vi "All_Stages_Action.vi"(6 "Positions":dbl[](array[numeric]), 8 "Axis":bool[](array[boolean]), 9 "Action":T1=enum."MVR", 10 "Stage ID":string, 11 "State Cluster":T2={"Stages"={"M686"={"VISA"="", "Status"=FALSE, "Positions"=[], "SpecialFunction"="", "ID"="M686"}, "P541"={"VISA"="", "Status"=FALSE, "Positions"=[], "SpecialFunction"="", "ID"="P541"}, "M227"={"VISA"="", "Status"=FALSE, "Positions"=[], "SpecialFunction"="", "ID"="M227"}, "N664"={"VISA"="", "Status"=FALSE, "Positions"=[], "SpecialFunction"="", "ID"="N664"}, "P612"={"VISA"="", "Status"=FALSE, "Positions"=[], "SpecialFunction"="", "ID"="P612"}, "ASI"={"VISA"="", "Status"=FALSE, "Positions"=[], "SpecialFunction"="", "ID"="ASI"}}, "Lasers"={"405"={"VISA"=""}, "561"={"handle"=0, "Return Value"=0}}}) -> (0 "Position Out":dbl[](array[numeric]), 3 "State Cluster Out":T2={"Stages"={"M686"={"VISA"="", "Status"=FALSE, "Positions"=[], "SpecialFunction"="", "ID"="M686"}, "P541"={"VISA"="", "Status"=FALSE, "Positions"=[], "SpecialFunction"="", "ID"="P541"}, "M227"={"VISA"="", "Status"=FALSE, "Positions"=[], "SpecialFunction"="", "ID"="M227"}, "N664"={"VISA"="", "Status"=FALSE, "Positions"=[], "SpecialFunction"="", "ID"="N664"}, "P612"={"VISA"="", "Status"=FALSE, "Positions"=[], "SpecialFunction"="", "ID"="P612"}, "ASI"={"VISA"="", "Status"=FALSE, "Positions"=[], "SpecialFunction"="", "ID"="ASI"}}, "Lasers"={"405"={"VISA"=""}, "561"={"handle"=0, "Return Value"=0}}})   [LabVIEW 2014]
uses:
  Controls/State_Cluster.ctl
  iPALM Control/Controls/StageStates.ctl
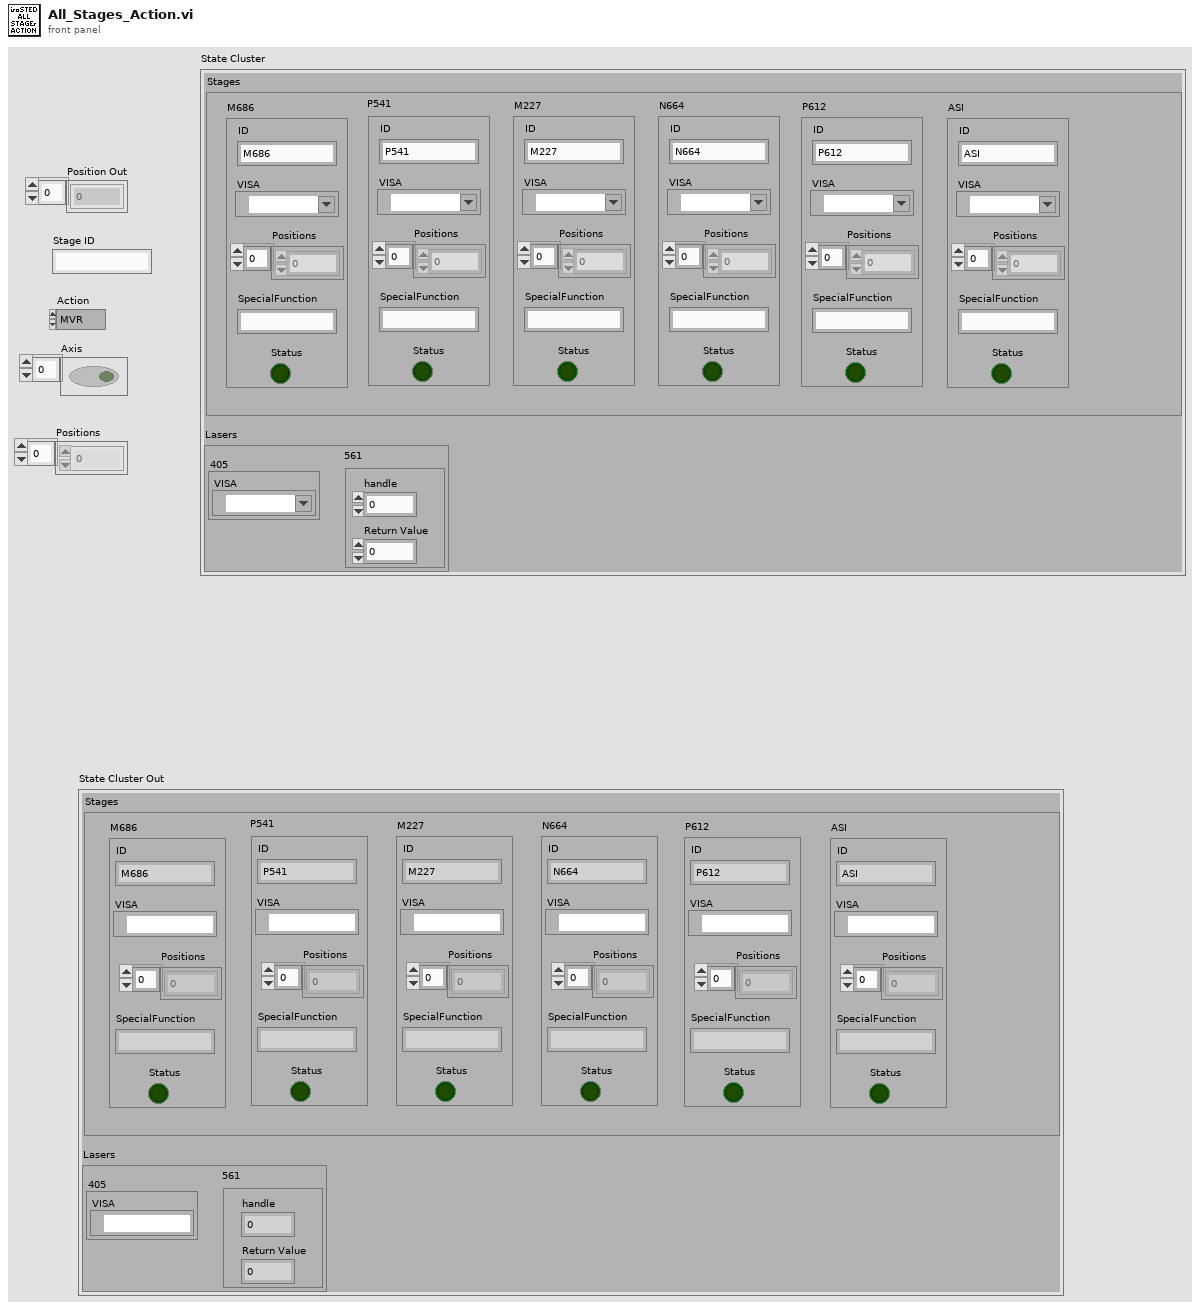
[diagram p1: front panel]
types:
  T1 = typedef "StageStates.ctl" = enum16{"POSITION", "MVR", "MOVE", "HALT", "ONTARGET", "ERROR", "EXIT", "HOME", "ZEROPOS", "NANOPOS", "QUIT", "ANALOG"}
  T2 = typedef "State_Cluster.ctl" = cluster{"Stages":cluster{"M686":cluster{"VISA":refnum<visa-resource-name>, "Status":bool, "Positions":dbl[], "SpecialFunction":string, "ID":string}, "P541":cluster{"VISA":refnum<visa-resource-name>, "Status":bool, "Positions":dbl[], "SpecialFunction":string, "ID":string}, "M227":cluster{"VISA":refnum<visa-resource-name>, "Status":bool, "Positions":dbl[], "SpecialFunction":string, "ID":string}, "N664":cluster{"VISA":refnum<visa-resource-name>, "Status":bool, "Positions":dbl[], "SpecialFunction":string, "ID":string}, "P612":cluster{"VISA":refnum<visa-resource-name>, "Status":bool, "Positions":dbl[], "SpecialFunction":string, "ID":string}, "ASI":cluster{"VISA":refnum<visa-resource-name>, "Status":bool, "Positions":dbl[], "SpecialFunction":string, "ID":string}}, "Lasers":cluster{"405":cluster{"VISA":refnum<visa-resource-name>}, "561":cluster{"handle":u32, "Return Value":i32}}}
  T3 = cluster{"M686":cluster{"VISA":refnum<visa-resource-name>, "Status":bool, "Positions":dbl[], "SpecialFunction":string, "ID":string}, "P541":cluster{"VISA":refnum<visa-resource-name>, "Status":bool, "Positions":dbl[], "SpecialFunction":string, "ID":string}, "M227":cluster{"VISA":refnum<visa-resource-name>, "Status":bool, "Positions":dbl[], "SpecialFunction":string, "ID":string}, "N664":cluster{"VISA":refnum<visa-resource-name>, "Status":bool, "Positions":dbl[], "SpecialFunction":string, "ID":string}, "P612":cluster{"VISA":refnum<visa-resource-name>, "Status":bool, "Positions":dbl[], "SpecialFunction":string, "ID":string}, "ASI":cluster{"VISA":refnum<visa-resource-name>, "Status":bool, "Positions":dbl[], "SpecialFunction":string, "ID":string}}
  T4 = cluster{"VISA":refnum<visa-resource-name>, "Status":bool, "Positions":dbl[], "SpecialFunction":string, "ID":string}[]
  T5 = cluster{"VISA":refnum<visa-resource-name>, "Status":bool, "Positions":dbl[], "SpecialFunction":string, "ID":string}
  T6 = cluster{"Stages[0]":cluster{"VISA":refnum<visa-resource-name>, "Status":bool, "Positions":dbl[], "SpecialFunction":string, "ID":string}, "Stages[1]":cluster{"VISA":refnum<visa-resource-name>, "Status":bool, "Positions":dbl[], "SpecialFunction":string, "ID":string}, "Stages[2]":cluster{"VISA":refnum<visa-resource-name>, "Status":bool, "Positions":dbl[], "SpecialFunction":string, "ID":string}, "Stages[3]":cluster{"VISA":refnum<visa-resource-name>, "Status":bool, "Positions":dbl[], "SpecialFunction":string, "ID":string}, "Stages[4]":cluster{"VISA":refnum<visa-resource-name>, "Status":bool, "Positions":dbl[], "SpecialFunction":string, "ID":string}, "Stages[5]":cluster{"VISA":refnum<visa-resource-name>, "Status":bool, "Positions":dbl[], "SpecialFunction":string, "ID":string}}
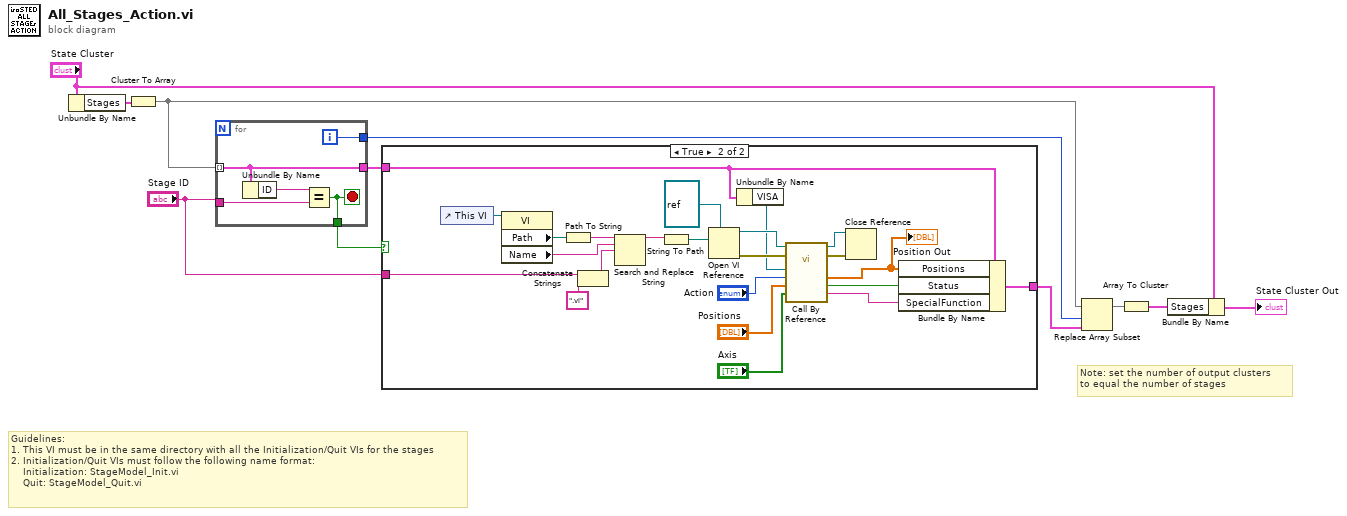
[diagram p0: block diagram]
diagram:
  # "Note: set the number of output clusters \nto equal the number of stages"
  # "Guidelines:\n1. This VI must be in the same directory with all the Initialization/Quit VIs for the stages\n2. Initialization/Quit VIs must follow the following name format:\n    Initialization: StageModel_Init.vi\n    Quit: StageModel_Quit.vi"
  n1 = Unbundle By Name("State Cluster") -> ("Stages"=w4:T3)
  n2 = Cluster To Array(cluster=w4) -> (array=w11:T4)
  n3 = for {
    tunnel: w11 -> [w15] mode=indexing
    tunnel: "Stage ID" -> [w16]
    tunnel: [w15] -> w6
    tunnel: [w14] -> w10
    tunnel: [w12] -> w7
    i -> [w14]
    stop <- w12 stop-if-true
    n4 = Unbundle By Name(w15) -> ("ID"=w13:string)
    n5 = Equal?(x=w13, y=w16) -> (x = y?=w12:bool)
  }
  n6 = case shown="True" w7 {
    tunnel: [w17 w35] -> w5
    tunnel: "Stage ID" -> [_ w36]
    tunnel: w6 -> [w17 w22]
    frame False {
    }
    frame True {
      n7 = control-ref of="This VI"() -> (w40:refnum<vi>)
      n8 = property class="VI"(reference=w40) -> ("Path"=w39:path, "Name"=w37:string)  [unwired: 1 in, 2 out]
      n9 = Path To String(path=w39) -> (string=w38:string)
      n10 = Concatenate Strings(w36, ".vi" ("string")) -> (w25:string)
      n11 = Search and Replace String(input string=w38, search string=w37, replace string=w25) -> (result string=w32:string)  [unwired: 5 in, 3 out]
      n12 = String To Path(string=w32) -> (path=w31:path)
      n13 = Open VI Reference(type specifier VI Refnum (for type only)=refnum<vi> refnum, vi path=w31) -> (vi reference=w29:refnum<vi>, error out=w27:errorcluster)  [unwired: 4 in]
      n14 = Unbundle By Name(w22) -> ("VISA"=w20:refnum<visa-resource-name>)
      n15 = call-by-ref "?"(reference=w29, error in=w27, "Axis"="Axis", "Positions In"="Positions", "Action"="Action", "VISA In"=w20) -> (reference out=w28:refnum<vi>, error out=w26:errorcluster, "Special Function Out"=w23:string, "Status"=w33:bool, "Position Out"=w34:dbl[])  [unwired: 4 in, 1 out]
      "Position Out" <- w34
      n16 = Close Reference(reference=w28, error in (no error)=w26) -> ()  [unwired: 1 out]
      n17 = Bundle By Name(cluster=w22, "Positions"=w34, "Status"=w33, "SpecialFunction"=w23) -> (w35:T5)
    }
  }
  n18 = Replace Array Subset(array=w11, new element=w5, index=w10) -> (w8:T4)
  n19 = Array To Cluster(array=w8) -> (cluster=w2:T6)
  n20 = Bundle By Name(cluster="State Cluster", "Stages"=w2) -> (→"State Cluster Out":T2)
